vi "VISA Test.vi"(8 "error in":errorcluster, 10 "Command":string, 11 "VISA resource name":refnum<visa-resource-name>) -> (0 "error out":errorcluster, 2 "Instrument Response":string, 3 "VISA resource name out":refnum<visa-resource-name>)   [LabVIEW 2020, in "Omega Platinum Series.lvlib"]
doc: "Simple VI designed to test VISA communication to the instrument. This application opens a session to the instrument, performs a write of the fetch ID command \"ID\\r\", and queries the device for its response."
uses:
  <instrlib>/RxnRover/OmegaPlatinumSeriesDriver/Omega Platinum Series.lvlib
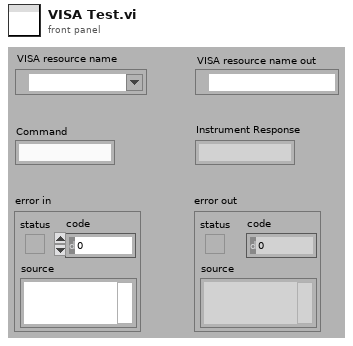
[diagram p1: front panel]
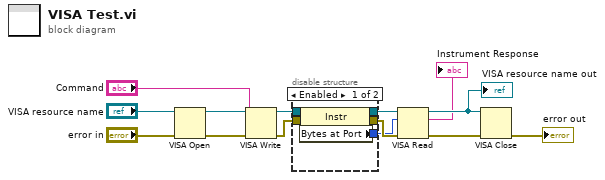
[diagram p0: block diagram]
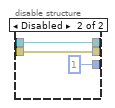
[diagram p2: hidden frame]
diagram:
  n1 = VISA Open(error in (no error)="error in", VISA resource name="VISA resource name") -> (VISA resource name=w12:refnum<visa-resource-name>, error out=w11:errorcluster)  [unwired: 3 in]
  n2 = VISA Write(VISA resource name=w12, write buffer="Command", error in (no error)=w11) -> (VISA resource name out=w6:refnum<visa-resource-name>, error out=w4:errorcluster)  [unwired: 1 out]
  n3 = disable-structure shown="Enabled" {
    disable-tunnel: w6 -> [w19 w22]
    disable-tunnel: [w18 w22] -> w5
    disable-tunnel: w4 -> [w17 w21]
    disable-tunnel: [w16 w21] -> w3
    disable-tunnel: [w15 1] -> w2
    frame Enabled {
      n4 = property class="Instr"(reference=w19, error in=w17) -> (reference out=w18:refnum<visa-resource-name>, error out=w16:errorcluster, "Bytes at Port"=w15:u32)
    }
    frame Disabled {
    }
  }
  n5 = VISA Read(VISA resource name=w5, byte count=w2, error in (no error)=w3) -> (VISA resource name out=w8:refnum<visa-resource-name>, read buffer=→"Instrument Response":string, error out=w10:errorcluster)  [unwired: 1 out]
  "VISA resource name out" <- w8
  n6 = VISA Close(VISA resource name=w8, error in (no error)=w10) -> (error out=→"error out":errorcluster)
